vi "MockHPILC.vi"(11 "MockHPILCSettings":T1={"ModbusRxDataFIFO"="MockbusPort2RxFIFO", "ModbusTxDataFIFO"="ModbusPort2TxInternalFIFO", "BufferUpdateFIFO"="MockHPILCCommand", "Code17Memory"="MockHPILCCode17", "Code18Memory"="MockHPILCCode18", "Code65Memory"="MockHPILCCode65", "Code66Memory"="MockHPILCCode66", "Code67Memory"="MockHPILCCode67", "Code72Memory"="MockHPILCCode72", "Code80Memory"="MockHPILCCode80", "Code110Memory"="MockHPILCCode110"}) -> ()   [LabVIEW 2016, in "FPGAMockMDILC.lvlib"]
uses:
  FPGAMockMDILC.lvlib
  DataTypes/MockHPILCSettings.ctl
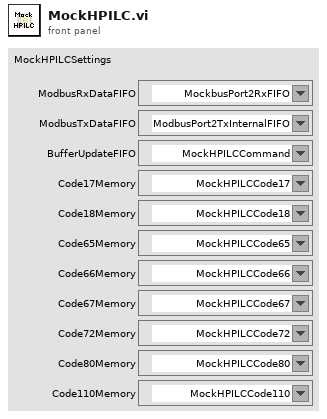
[diagram p1: front panel]
types:
  T1 = typedef "FPGAMockMDILC.lvlib/MockHPILCSettings.ctl" = cluster{"ModbusRxDataFIFO":refnum<k21>, "ModbusTxDataFIFO":refnum<k21>, "BufferUpdateFIFO":refnum<k21>, "Code17Memory":refnum<k21>, "Code18Memory":refnum<k21>, "Code65Memory":refnum<k21>, "Code66Memory":refnum<k21>, "Code67Memory":refnum<k21>, "Code72Memory":refnum<k21>, "Code80Memory":refnum<k21>, "Code110Memory":refnum<k21>}
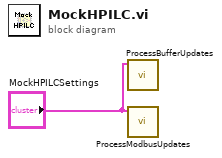
[diagram p0: block diagram]
diagram:
  n1 = call "ProcessBufferUpdates.vi"("MockHPILCSettings"="MockHPILCSettings") -> ()  [unwired: 11 in]
  n2 = call "ProcessModbusUpdates.vi"("MockHPILCSettings"="MockHPILCSettings") -> ()  [unwired: 11 in]
